vi "PruebaAutoRefresh.vi"() -> ()   [LabVIEW 2014, in "MSX-E3711.lvlib"]
uses:
  MSX-E3711Class/MSX-E3711.lvlib
  DriverMasterSync/build/DriverMasterSync.lvlibp/APIs/Data Queue/Control Data Cluster.ctl
  DriverMasterSync/build/DriverMasterSync.lvlibp/APIs/Data Queue/Acquisition Data 1 Sample Cluster.ctl
  DriverMasterSync/build/DriverMasterSync.lvlibp/Modules/HAL/TypeDefs/HAL Config Data.ctl
  MSX-E3711Class/MSX-E3711.lvclass
  DriverMasterSync/build/DriverMasterSync.lvlibp/APIs/Data Queue/WINFAS 2 Data Queue.lvlib
  DriverMasterSync/build/DriverMasterSync.lvlibp
panel:
  out "HAL Config Data":T1
  in  "PromCycle":bool
  out "1 Sample":T2
  out "Control Data":T3
  in  "stop":bool
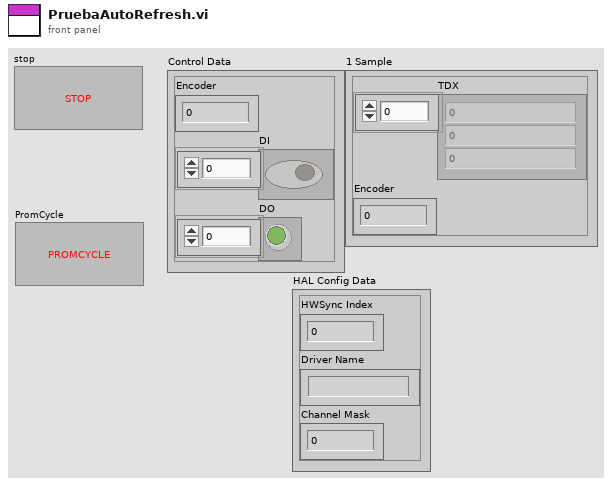
[diagram p1: front panel]
types:
  T1 = typedef "DriverMasterSync.lvlibp/HAL Config Data.ctl" = cluster{"HWSync Index":u32, "Driver Name":string, "Channel Mask":u64}
  T2 = typedef "DriverMasterSync.lvlibp/WINFAS 2 Data Queue.lvlib/Acquisition Data 1 Sample Cluster.ctl" = cluster{"TDX":sgl[], "Encoder":sgl}
  T3 = typedef "DriverMasterSync.lvlibp/WINFAS 2 Data Queue.lvlib/Control Data Cluster.ctl" = cluster{"Encoder":sgl, "DI":bool[], "DO":bool[]}
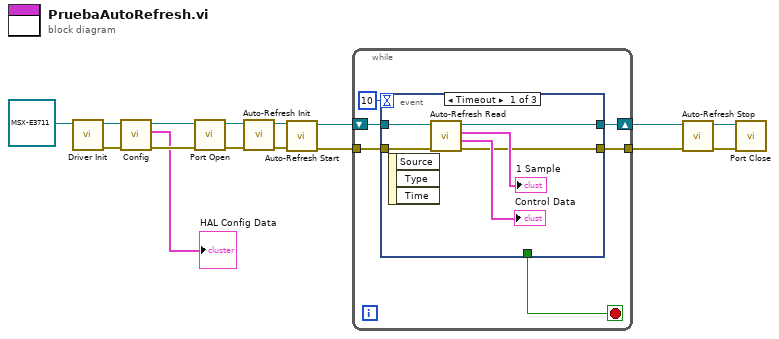
[diagram p0: block diagram]
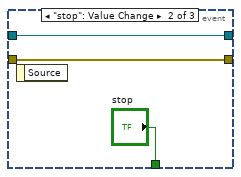
[diagram p2: hidden frame]
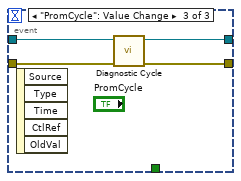
[diagram p3: hidden frame]
diagram:
  n1 = call-dynamic "Driver Init.vi"("MSX-E3711 in"=refnum<class "MSX-E3711.lvclass"> refnum) -> ("error out"=w1:errorcluster, "MSX-E3711 out"=w3:refnum<class "MSX-E3711.lvclass">)  [unwired: 9 in]
  n2 = call-dynamic "Config.vi"("error in (no error)"=w1, "MSX-E3711 in"=w3) -> ("error out"=w8:errorcluster, "HAL Config Data"=→"HAL Config Data":T1, "MSX-E3711 out"=w9:refnum<class "MSX-E3711.lvclass">)  [unwired: 7 in]
  n3 = call-dynamic "Port Open.vi"("error in (no error)"=w8, "MSX-E3711 in"=w9) -> ("error out"=w6:errorcluster, "MSX-E3711 out"=w7:refnum<class "MSX-E3711.lvclass">)  [unwired: 8 in]
  n4 = call-dynamic "Auto-Refresh Init.vi"("error in (no error)"=w6, "MSX-E3711 in"=w7) -> ("error out"=w12:errorcluster, "MSX-E3711 out"=w4:refnum<class "MSX-E3711.lvclass">)  [unwired: 8 in]
  n5 = call-dynamic "Auto-Refresh Start.vi"("error in (no error)"=w12, "MSX-E3711 in"=w4) -> ("error out"=w10:errorcluster, "MSX-E3711 out"=w11:refnum<class "MSX-E3711.lvclass">)  [unwired: 8 in]
  n6 = while {
    tunnel: w10 -> [w17]
    tunnel: [w20] -> w14
    shift-right: [w21] -> w16
    shift-left: w11 -> [w22]
    stop <- w19 stop-if-true
    n7 = event shown="[0] Timeout" {
      selector: _ -> [_ _ _]
      dyn-events: _ -> [_ _ _]
      timeout: 10 -> [_ _ _]
      tunnel: w22 -> [w28 w29 w35]
      tunnel: w17 -> [w27 w30 w32]
      tunnel: [w26 w29 w34] -> w21
      tunnel: [w23 w30 w33] -> w20
      tunnel: [_ "stop" _] -> w19
      event Timeout {
        n8 = event-data() -> ()  [unwired: 1 in, 3 out]
        n9 = call-dynamic "Auto-Refresh Read.vi"("error in (no error)"=w27, "MSX-E3711 in"=w28) -> ("error out"=w23:errorcluster, "Control Data"=→"Control Data":T3, "1 Sample"=→"1 Sample":T2, "MSX-E3711 out"=w26:refnum<class "MSX-E3711.lvclass">)  [unwired: 6 in]
      }
      event "stop": Value Change {
        n10 = event-data() -> ()  [unwired: 1 in, 1 out]
      }
      event "PromCycle": Value Change {
        n11 = event-data() -> ()  [unwired: 1 in, 5 out]
        n12 = call-dynamic "Diagnostic Cycle.vi"("error in (no error)"=w32, "MSX-E3711 in"=w35) -> ("error out"=w33:errorcluster, "MSX-E3711 out"=w34:refnum<class "MSX-E3711.lvclass">)  [unwired: 8 in]
      }
    }
  }
  n13 = call-dynamic "Auto-Refresh Stop.vi"("error in (no error)"=w14, "MSX-E3711 in"=w16) -> ("error out"=w13:errorcluster, "MSX-E3711 out"=w15:refnum<class "MSX-E3711.lvclass">)  [unwired: 8 in]
  n14 = call-dynamic "Port Close.vi"("error in (no error)"=w13, "MSX-E3711 in"=w15) -> ()  [unwired: 8 in, 2 out]
